vi "readTriggerLevelWindow.vi"(8 "error in (no error)":errorcluster, 10 "output cluster in":T1={"DC Restore"=enum."off", "Polarity"=enum."Negative", "TV Event"=enum."Field 1", "Coupling"=enum."AC", "Slope"=enum."Negative", "AnalogSource"=enum."Channel 0", "Window Mode"=enum."Entering", "Low Level"=0.0, "High Level"=0.0, "Hysteresis"=0.0, "Delay"=0.0, "Holdoff"=0.0, "Signal Format"=enum."M-NTSC", "Mode"=enum."Immediate", "Line Number"=0, "DigitalSource"=enum."RTSI 0"}, 11 "IVI Refnum in":refnum<k15>) -> (0 "error out":errorcluster, 2 "output cluster out":T1={"DC Restore"=enum."off", "Polarity"=enum."Negative", "TV Event"=enum."Field 1", "Coupling"=enum."AC", "Slope"=enum."Negative", "AnalogSource"=enum."Channel 0", "Window Mode"=enum."Entering", "Low Level"=0.0, "High Level"=0.0, "Hysteresis"=0.0, "Delay"=0.0, "Holdoff"=0.0, "Signal Format"=enum."M-NTSC", "Mode"=enum."Immediate", "Line Number"=0, "DigitalSource"=enum."RTSI 0"}, 3 "IVI Refnum out":refnum<k15>)   [LabVIEW 2011]
uses:
  TriggerSettings_TypDef.ctl
  OnOffTypeDef.ctl
  Polarity_TypDEf.ctl
  TVEvent_TypDef.ctl
  coupling_TypDef.ctl
  positive_negatice2_typDef.ctl
  TriggerSource_TypDef.ctl
  triggerwindowmode2_TypDef.ctl
  SignalFormat_TypDef.ctl
  mode_TypDef.ctl
  Trigger.DigitalSource_TypDEf.ctl
panel:
  out "Triggering:Trigger Source":string
  out "Triggering:Trigger Level":dbl
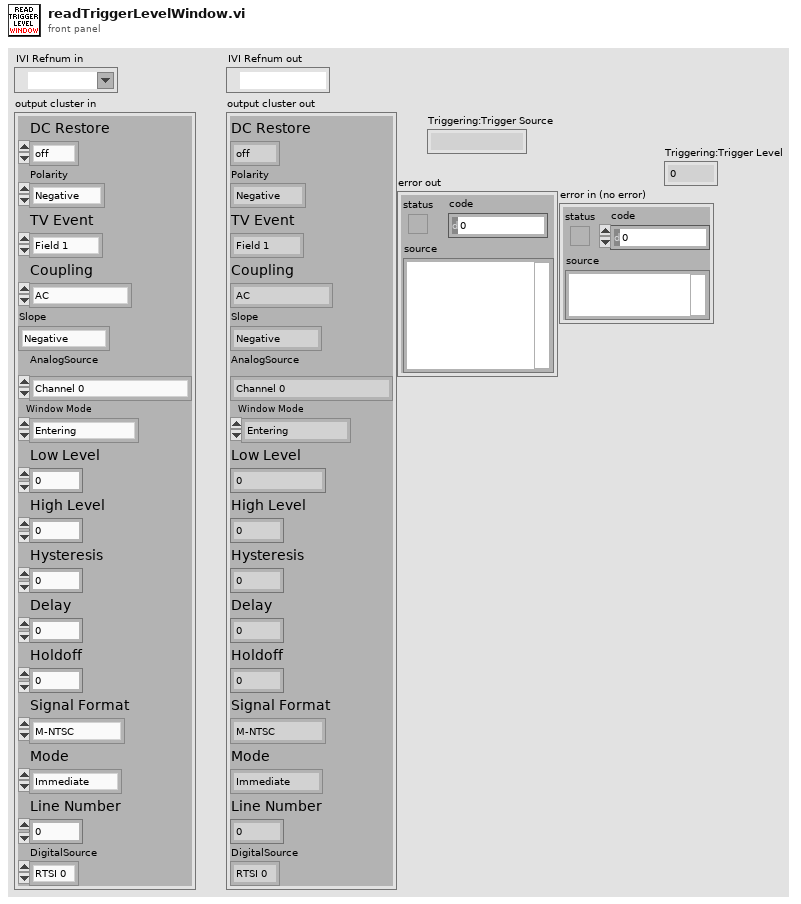
[diagram p1: front panel]
types:
  T1 = typedef "TriggerSettings_TypDef.ctl" = cluster{"DC Restore":T2, "Polarity":T3, "TV Event":T4, "Coupling":T5, "Slope":T6, "AnalogSource":T7, "Window Mode":T8, "Low Level":dbl, "High Level":dbl, "Hysteresis":dbl, "Delay":dbl, "Holdoff":dbl, "Signal Format":T9, "Mode":T10, "Line Number":i32, "DigitalSource":T11}
  T2 = typedef "OnOffTypeDef.ctl" = enum16{"off", "on"}
  T3 = typedef "Polarity_TypDEf.ctl" = enum16{"Negative", "Positive"}
  T4 = typedef "TVEvent_TypDef.ctl" = enum16{"Field 1", "Field 2", "Any Field", "Any Line", "Line Number"}
  T5 = typedef "coupling_TypDef.ctl" = enum16{"AC", "DC", "HF Reject", "LF Reject", "AC Plus HF Reject"}
  T6 = typedef "positive_negatice2_typDef.ctl" = enum16{"Positive", "Negative"}
  T7 = typedef "TriggerSource_TypDef.ctl" = enum16{"Channel 0", "Channel 1", "External TRIG"}
  T8 = typedef "triggerwindowmode2_TypDef.ctl" = enum16{"Entering", "Leaving"}
  T9 = typedef "SignalFormat_TypDef.ctl" = enum16{"M-NTSC", "B/G-PAL", "SECAM", "M-PAL", "480i/59.94 fps", "480i/60 fps", "480p/59.94 Fps", "480p/60 Fps", "576i/50 fps", "576p/50 Fps", "720p/50 Fps", "720p/59.94 Fps", "720p/60 Fps", "1080i/50 fps", "1080i/59.94 fps", "1080i/60 fps", "1080p/24 Fps"}
  T10 = typedef "mode_TypDef.ctl" = enum32{"Immediate", "Analog Edge", "Analog Window", "Analog Hysteresis", "Video", "Digital Edge"}
  T11 = typedef "Trigger.DigitalSource_TypDEf.ctl" = enum16{"RTSI 0", "RTSI 1", "RTSI 2", "RTSI 3", "RTSI 4", "RTSI 5", "RTSI 6", "PFI 0", "PFI 1", "PFI 2", "PXI Star Trigger"}
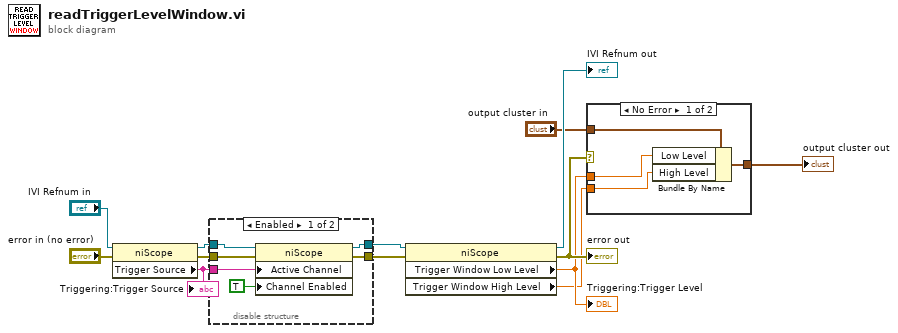
[diagram p0: block diagram]
diagram:
  n1 = property class="niScope"(reference="IVI Refnum in", error in="error in (no error)") -> (reference out=w11:refnum<k15>, error out=w6:errorcluster, "Trigger Source"=w10:string)
  "Triggering:Trigger Source" <- w10
  n2 = disable-structure shown="Enabled" {
    disable-tunnel: w11 -> [w19 w21]
    disable-tunnel: [w18 w21] -> w9
    disable-tunnel: w10 -> [w17 _]
    disable-tunnel: [w16 w20] -> w7
    disable-tunnel: w6 -> [w15 w20]
    frame Enabled {
      n3 = property class="niScope"(reference=w19, error in=w15, "Active Channel"=w17, "Channel Enabled"=TRUE ("Vertical:Channel Enabled")) -> (reference out=w18:refnum<k15>, error out=w16:errorcluster)
    }
    frame Disabled {
    }
  }
  n4 = property class="niScope"(reference=w9, error in=w7) -> (reference out=→"IVI Refnum out":refnum<k15>, error out=w4:errorcluster, "Trigger Window Low Level"=w3:dbl, "Trigger Window High Level"=w1:dbl)
  "error out" <- w4
  "Triggering:Trigger Level" <- w3
  n5 = case shown="No Error" w4 {
    tunnel: [w25 w26] -> w13
    tunnel: "output cluster in" -> [w24 w26]
    tunnel: w3 -> [w23 _]
    tunnel: w1 -> [w22 _]
    frame No Error {
      n6 = Bundle By Name(cluster=w24, "Low Level"=w23, "High Level"=w22) -> (w25:T1)
    }
    frame Error {
    }
  }
  "output cluster out" <- w13
